vi "2023_day08_Task2.vi"() -> ()   [LabVIEW 2021]
panel:
  out "Task 2":u64
  in  "Switch":bool caption="Ex. Data  vs.  User Data"
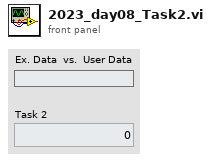
[diagram p1: front panel]
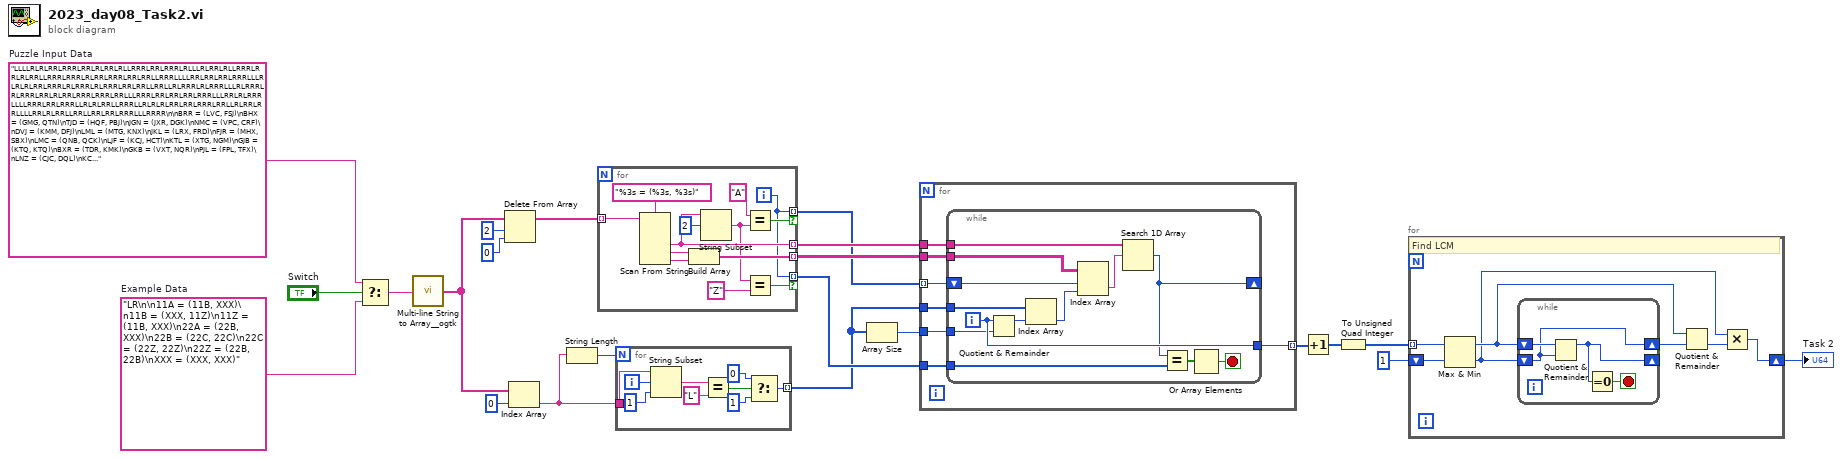
[diagram p0: block diagram]
diagram:
  w21 = "LLLLRLRLRRLRRRLRRLRLRRLRLLRRRLRRLRRRLRLLLRLRRLRLLRRRLRRLRLRRLLRRRLRRRLRLRRLRRRLRRLRRLLRRRLLLLRRLRRLRRLRRRLLLRLRLRLRRLRRRLRLRRRLRLRRRLRRLRRLLRRLLRLRRRLRLRRRLLLRLRRRLRLRRRLRRLRLRRLRRRLRRRLRRLLLRRRLRRLRRLRRLRRRLLLRRLRLRRRLLLLRRRLRRLRRRLLRLRLRRLLRRRLLRLRLRLRRLRRLRRRLRRLLRLRRLRRLLLLRRLRLRRLLRRLLRRLRRLRRRLLLRRRR\n\nBRR = (LVC, FSJ)\nBHX = (GMG, QTN)\nTJD = (HQF, PBJ)\nJGN = (JXR, DGK)\nNMC = (VPC, CRF)\nDVJ = (KMM, DFJ)\nLML = (MTG, KNX)\nJKL = (LRX, FRD)\nFJR = (MHX, SBX)\nLMC = (QNB, QCK)\nLJF = (KCJ, HCT)\nKTL = (XTG, NGM)\nGJB = (KTQ, KTQ)\nBXR = (TDR, KMK)\nGKB = (VXT, NQR)\nPJL = (FPL, TFX)\nLNZ = (CJC, DQL)\nKCG = (KDL, LMF)\nPGG = (NDL, XXC)\nPMS = (XQM, DFG)\nCJF = (MCG, RTJ)\nJTH = (PGS, SGZ)\nQBS = (JSC, KMT)\nDQL = (KRR, PBL)\nHSF = (SNP, KJR)\nXVQ = (VQR, HSX)\nQKF = (PBT, XLC)\nDNA = (DQL, CJC)\nLNF = (RVC, TJD)\nMKT = (LDX, CGC)\nBXP = (RGX, TTR)\nSBX = (PGT, JGN)\nJQK = (HDQ, BHQ)\nMHL = (TLX, JDN)\nBBD = (QNJ, BRM)\nMTT = (BVK, DXB)\nFVR = (VLN, PRV)\nRVC = (HQF, PBJ)\nLDX = (LRS, KBV)\nBKF = (PXH, TNB)\nBRM = (XTV, NGH)\nDDL = (JNG, SFF)\nBBT = (BQJ, BCN)\nGPK = (CVK, DDL)\nTLX = (BDN, XNT)\nJHL = (BRX, QBT)\nNTL = (HSR, DJD)\nXBH = (PJX, JQK)\nPPF = (LCT, BJL)\nSFF = (FVR, NFG)\nHNA = (CTC, BSG)\nCNG = (DXM, QFN)\nGML = (NRD, TVN)\nRHH = (NBT, LJH)\nLDM = (DDN, TRN)\nXSK = (PLB, NVJ)\nNCQ = (MDN, XGT)\nFCQ = (HCT, KCJ)\nDRC = (JKL, JNM)\nSHR = (KLX, VLH)\nFTP = (DRN, DKV)\nQBF = (GVS, NXK)\nGXK = (XDK, LVF)\nKMK = (VXV, XCS)\nPKK = (QNJ, BRM)\nNJH = (TKL, PQK)\nBRX = (MNM, HVC)\nVTD = (BJK, LML)\nQVX = (DVJ, DSF)\nGRM = (JCV, SQB)\nRDQ = (HCG, XMB)\nRGX = (FCN, TPD)\nHBH = (FPR, DHX)\nPHM = (JSP, RCR)\nNBT = (FRG, CMJ)\nXRH = (HCB, FBM)\nGMR = (FDJ, NJD)\nMVG = (RDJ, QSD)\nBDL = (JSB, TFN)\nVXT = (MBM, JND)\nTXC = (QDG, LTV)\nSRL = (RRX, NDS)\nSGN = (MPL, CBB)\nHVH = (SLJ, CBC)\nVPC = (CCG, QSJ)\nKCJ = (CKC, TTD)\nRLT = (LLT, VVL)\nRXV = (KXQ, VBR)\nFQS = (STP, BHX)\nSGC = (RLJ, QGB)\nXLX = (HRG, DGV)\nXKV = (QQB, TNQ)\nSLJ = (GTB, MPF)\nPKV = (CQN, THS)\nRPP = (QFT, TNK)\nDKL = (MFC, MFC)\nBCG = (FXM, GPR)\nRFV = (DRC, MPD)\nVVC = (FGN, CVL)\nHQB = (QNT, VVC)\nRRP = (VVC, QNT)\nTRS = (RCM, GHN)\nQBT = (HVC, MNM)\nXKS = (SCC, VXX)\nTPS = (FMH, KFN)\nMTS = (VXT, NQR)\nFXM = (LDM, FQT)\nLNB = (XJV, SJN)\nHVF = (QXC, RBH)\nLSG = (QHM, TSM)\nJMP = (HBH, NQK)\nNGM = (KDP, HHP)\nHCG = (SLR, TSC)\nHGX = (DFG, XQM)\nDLG = (BVN, GMM)\nDJD = (VGP, VML)\nHBT = (XKL, JBQ)\nNVJ = (GKX, PKS)\nCPS = (PKJ, RSV)\nSKN = (NBT, LJH)\nCCK = (TTJ, SLV)\nDXM = (CBN, BXR)\nRJD = (XJH, SKH)\nRDJ = (CNF, TTG)\nPKJ = (BCM, XKC)\nFQL = (SRV, DFC)\nKDS = (MFB, CLQ)\nQKR = (VGD, CXK)\nXXC = (NFD, SPS)\nPSQ = (NJH, BLR)\nBLR = (PQK, TKL)\nLMX = (DGV, HRG)\nGCK = (CSR, CSR)\nGKJ = (JHL, PNN)\nGVS = (TLN, LJX)\nFPR = (JCH, GKD)\nVQV = (DGB, GGN)\nCPF = (VMH, JQQ)\nGKD = (SGF, PHM)\nJNM = (LRX, FRD)\nCXV = (LNF, HGF)\nTNK = (RRD, HKC)\nDXX = (LMC, ZZZ)\nDGG = (PPF, TRR)\nMLH = (TVL, PBR)\nLBC = (LJL, FTR)\nFVQ = (TBC, LKB)\nLTF = (CBC, SLJ)\nTVH = (XMS, GJS)\nSFB = (TTJ, SLV)\nLVF = (MBT, SJB)\nXPP = (QDM, PJL)\nBVK = (RPV, JMP)\nVGD = (MRX, FJR)\nFRD = (XBH, CDN)\nLKM = (CMF, XNS)\nTCJ = (MMS, PGG)\nDHQ = (MTT, BKS)\nHDQ = (GPH, XKH)\nKTJ = (QQT, MKR)\nNMQ = (VFK, VSD)\nRSK = (QDM, PJL)\nXQC = (KFP, HVB)\nLQN = (NGM, XTG)\nTKG = (XDQ, XDQ)\nKBB = (VQR, HSX)\nTQQ = (QDG, LTV)\nSQN = (TDQ, XKV)\nTSM = (TSH, MRP)\nKPH = (THS, CQN)\nHCB = (DVL, RTV)\nMLR = (GHT, NSN)\nBFM = (GCK, SLX)\nGXQ = (QKM, JJL)\nGNF = (HRQ, XTK)\nTRR = (BJL, LCT)\nAAA = (QNB, QCK)\nSDL = (KJX, LSN)\nDKV = (KBB, XVQ)\nRMR = (MQR, CPR)\nMQC = (CBV, SRP)\nPRV = (KDS, FBX)\nGTB = (CCK, SFB)\nSNP = (PXX, SHR)\nNTR = (VHT, KXK)\nMKJ = (DDL, CVK)\nLSQ = (HSF, RMN)\nTTJ = (CBH, QKF)\nDNH = (MVG, JCJ)\nKMM = (KPH, PKV)\nNTT = (RQK, PFK)\nQMF = (BFM, PJB)\nRJB = (RBH, QXC)\nLRS = (MJT, BVM)\nCJG = (RMR, BMN)\nDVQ = (GXM, DDH)\nMFC = (LMC, LMC)\nXTG = (HHP, KDP)\nHKB = (RDQ, TVT)\nPKS = (JQM, DGG)\nBJK = (KNX, MTG)\nTVT = (XMB, HCG)\nJNR = (JHG, JLN)\nVFK = (XKS, QBH)\nNPC = (PKK, BBD)\nPXX = (KLX, VLH)\nXLC = (NST, BXP)\nCBB = (LMX, XLX)\nKLX = (MSH, LCF)\nCLQ = (JNF, JNC)\nTSS = (MKR, QQT)\nSSS = (RMQ, RCS)\nQSD = (TTG, CNF)\nNHG = (DVQ, VNB)\nCTC = (VCN, RJD)\nTHS = (QRH, GPT)\nKDR = (RTK, GKJ)\nNTD = (CGG, SPN)\nGHP = (NCQ, FCD)\nKXQ = (RLS, VRM)\nGNV = (BQJ, BCN)\nDXQ = (QHC, FXN)\nRQB = (FVQ, TNF)\nCNF = (TXC, TQQ)\nBGB = (QQS, LRV)\nZZZ = (QCK, QNB)\nNFM = (MGV, VTD)\nMFD = (DBF, KSN)\nNST = (RGX, TTR)\nXJV = (LGL, LGL)\nTRQ = (TVH, KJL)\nPPV = (CJP, VHH)\nDNV = (DBM, VGJ)\nJBQ = (MHL, RFN)\nHRG = (JFD, VQP)\nRMB = (JKJ, JGJ)\nRGQ = (RSK, XPP)\nKHF = (TJG, KPX)\nHPZ = (BSG, CTC)\nLFJ = (TSN, NMB)\nMBT = (XRC, PJR)\nQFN = (CBN, BXR)\nQSJ = (BRS, BKF)\nXJH = (RSF, VNP)\nGST = (LVF, XDK)\nDDN = (NMS, RLT)\nCXK = (FJR, MRX)\nPHH = (FPB, TCJ)\nXHV = (KTJ, TSS)\nVHT = (NPC, DMG)\nRNL = (NHG, DVN)\nTKL = (KPN, FKX)\nDGB = (GPJ, QMF)\nPNN = (QBT, BRX)\nTBC = (NTR, FKG)\nPGS = (QDT, JQL)\nSLX = (CSR, LNB)\nBVV = (LVC, FSJ)\nJQL = (MLH, GSC)\nPXH = (CJF, CKM)\nLHM = (DSF, DVJ)\nNND = (NTD, DTB)\nMFB = (JNF, JNC)\nTTR = (FCN, TPD)\nHRQ = (JTD, JTD)\nSLR = (TXT, JSN)\nVQP = (XPK, XGB)\nQHM = (MRP, TSH)\nRTJ = (PXB, TLP)\nQQT = (RRL, QHQ)\nCSR = (XJV, XJV)\nCJP = (CJG, HQQ)\nRMC = (MPD, DRC)\nXMS = (LXX, GPN)\nHSR = (VGP, VML)\nMNM = (VSS, QXR)\nSJN = (LGL, LNZ)\nKBV = (MJT, BVM)\nKFN = (NRC, VSG)\nJNC = (RHR, LFJ)\nMPF = (SFB, CCK)\nQVK = (GNK, BCG)\nNJD = (KCG, LDB)\nDBM = (MJG, MFD)\nNKF = (GGN, DGB)\nBCN = (JNR, MHK)\nGNK = (FXM, GPR)\nKMT = (HFC, CPS)\nFDJ = (KCG, LDB)\nLVD = (PHH, QDR)\nFCN = (VDP, MQC)\nQQB = (GJB, GJB)\nPLF = (JNL, HBT)\nQDM = (FPL, TFX)\nGXM = (CLD, NNL)\nMRV = (BCG, GNK)\nLKB = (NTR, FKG)\nTTG = (TQQ, TXC)\nGFD = (VSD, VFK)\nRCS = (KQQ, DNH)\nQXR = (FCQ, LJF)\nHMQ = (RJQ, FQL)\nVCN = (SKH, XJH)\nQQG = (HSR, DJD)\nHGF = (RVC, TJD)\nXMB = (TSC, SLR)\nPJB = (GCK, SLX)\nHFC = (RSV, PKJ)\nJJL = (GXK, GST)\nQTN = (JLV, SGX)\nKDP = (GNV, BBT)\nVRF = (TFN, JSB)\nGPN = (CPF, SRQ)\nTSC = (TXT, JSN)\nCRF = (QSJ, CCG)\nTNF = (TBC, LKB)\nVLH = (LCF, MSH)\nBCV = (JSC, KMT)\nNNL = (KVX, FQS)\nRVT = (HCB, FBM)\nQHC = (QKV, NCJ)\nVDP = (CBV, SRP)\nCBV = (VQV, NKF)\nCMF = (XHV, TPR)\nTRN = (RLT, NMS)\nJSB = (XTH, TRS)\nCFC = (TVT, RDQ)\nKDL = (TKG, TKG)\nTTD = (BBC, GHP)\nKJR = (PXX, SHR)\nMTV = (GVS, NXK)\nBVN = (KDR, PVP)\nDXB = (RPV, JMP)\nFSJ = (QPQ, GML)\nPBJ = (LQN, KTL)\nPXB = (BDL, VRF)\nNDS = (BGB, NGX)\nCBN = (KMK, TDR)\nNFG = (VLN, PRV)\nJTD = (PGS, PGS)\nMKR = (QHQ, RRL)\nJSN = (RFV, RMC)\nCVK = (SFF, JNG)\nFGN = (BVQ, XQC)\nHHF = (RPS, QQF)\nPLB = (PKS, GKX)\nBJB = (QMC, GPG)\nSTP = (QTN, GMG)\nDGK = (RKK, BVT)\nJJM = (VGD, CXK)\nLTS = (QPN, BCL)\nLVC = (QPQ, GML)\nQNB = (GJN, RVB)\nRBH = (HMQ, HPS)\nNQK = (DHX, FPR)\nMRP = (BDT, SGN)\nJQM = (TRR, PPF)\nTSH = (BDT, SGN)\nJLN = (JCC, FCB)\nBRP = (LDX, CGC)\nSJC = (HRQ, HRQ)\nLJL = (BVB, PPV)\nSPN = (SDL, VHM)\nSDM = (DDF, LTS)\nLJH = (FRG, CMJ)\nCMG = (MKD, JGT)\nGPR = (LDM, FQT)\nQPQ = (NRD, TVN)\nJCJ = (RDJ, QSD)\nHSX = (CMG, SHF)\nVML = (RMB, MHC)\nDHX = (JCH, GKD)\nMTG = (FPX, SPD)\nBDT = (MPL, CBB)\nCJC = (PBL, KRR)\nJLS = (LJL, FTR)\nHQF = (LQN, KTL)\nHQQ = (RMR, BMN)\nQMC = (RBP, PXD)\nRPV = (HBH, NQK)\nJHG = (JCC, FCB)\nTPD = (VDP, MQC)\nBHQ = (XKH, GPH)\nXKC = (HDD, GXR)\nRPS = (KJP, KJP)\nQNT = (CVL, FGN)\nJSC = (HFC, CPS)\nKXG = (DTB, NTD)\nCKM = (RTJ, MCG)\nFTD = (KPX, TJG)\nVSD = (XKS, QBH)\nMCG = (TLP, PXB)\nXKH = (HLP, CXV)\nTNB = (CJF, CKM)\nXTH = (RCM, GHN)\nDFN = (GMR, DSS)\nLMF = (TKG, XST)\nFMH = (NRC, VSG)\nXCS = (JTS, GRM)\nGVF = (NDS, RRX)\nCXM = (HGX, PMS)\nVRM = (XJT, DXQ)\nJLV = (QVX, LHM)\nJCH = (PHM, SGF)\nNMS = (VVL, LLT)\nBHS = (XJR, LKM)\nCKC = (BBC, GHP)\nCBH = (XLC, PBT)\nPRL = (QFT, TNK)\nSDF = (VTD, MGV)\nRVB = (MLR, XHT)\nGPT = (PLF, MJX)\nKRR = (RVT, XRH)\nGXR = (BVV, BRR)\nNSN = (RGQ, JMQ)\nKJX = (TCR, MSL)\nPHL = (TSM, QHM)\nMQR = (MTS, GKB)\nXDK = (SJB, MBT)\nNRC = (DGN, BJB)\nJQQ = (LBC, JLS)\nJTS = (JCV, SQB)\nRLJ = (JJM, QKR)\nDTB = (CGG, SPN)\nBRS = (PXH, TNB)\nSRV = (SPC, DNV)\nMNP = (JJL, QKM)\nKTQ = (XSK, XSK)\nFPX = (SJC, GNF)\nVBR = (VRM, RLS)\nKSN = (HQB, RRP)\nRJQ = (SRV, DFC)\nBKS = (BVK, DXB)\nBVB = (VHH, CJP)\nXTK = (JTD, JTH)\nPBT = (BXP, NST)\nPVP = (RTK, GKJ)\nQPN = (BCV, QBS)\nQQF = (KJP, HPZ)\nQRH = (PLF, MJX)\nGHS = (BKN, TPS)\nRCM = (MNP, GXQ)\nDCT = (DDF, LTS)\nJLC = (HGX, PMS)\nVNC = (XSK, CXZ)\nBQJ = (MHK, JNR)\nSHF = (JGT, MKD)\nFXN = (QKV, NCJ)\nFPB = (PGG, MMS)\nJGJ = (KXG, NND)\nVBM = (PSQ, QKN)\nGKX = (DGG, JQM)\nDSF = (KMM, DFJ)\nCMJ = (GPK, MKJ)\nNCJ = (SDM, DCT)\nMKD = (GQG, DHQ)\nCFZ = (RQB, SHH)\nRQK = (DKL, DKL)\nXGT = (HPQ, VRQ)\nSRP = (NKF, VQV)\nBSG = (VCN, RJD)\nXRC = (NFM, SDF)\nDVL = (SRL, GVF)\nHVB = (HXS, MLD)\nMPD = (JNM, JKL)\nJSP = (PHL, LSG)\nBCR = (XJR, LKM)\nPQK = (KPN, FKX)\nFCD = (XGT, MDN)\nMDL = (JLC, CXM)\nFBX = (CLQ, MFB)\nVNP = (RGM, GHS)\nHMK = (RMN, HSF)\nSJB = (PJR, XRC)\nJFD = (XPK, XGB)\nHHP = (GNV, BBT)\nTVN = (VBM, KJN)\nDMG = (PKK, BBD)\nRGM = (BKN, TPS)\nTRF = (KXQ, VBR)\nXHT = (NSN, GHT)\nDFJ = (KPH, PKV)\nKJP = (CTC, BSG)\nLLT = (NTS, LVD)\nRMN = (SNP, KJR)\nGSC = (TVL, PBR)\nRSV = (XKC, BCM)\nTLP = (VRF, BDL)\nGGN = (GPJ, QMF)\nXJR = (CMF, XNS)\nGQG = (BKS, MTT)\nJPN = (MRV, QVK)\nRSF = (RGM, GHS)\nQQS = (DLG, JPV)\nDGV = (VQP, JFD)\nJDN = (XNT, BDN)\nLMA = (QDT, JQL)\nQDG = (QGC, DTX)\nHDD = (BVV, BRR)\nRRD = (CNG, XLJ)\nQBH = (VXX, SCC)\nGPH = (HLP, CXV)\nCVN = (MRV, QVK)\nRLS = (XJT, DXQ)\nQKN = (NJH, BLR)\nNRD = (VBM, KJN)\nNMB = (HVF, RJB)\nXNT = (RXV, TRF)\nXNS = (XHV, TPR)\nSGX = (LHM, QVX)\nNTS = (PHH, QDR)\nSPS = (LTF, HVH)\nKPX = (BCR, BHS)\nGNM = (RPS, RPS)\nCXZ = (NVJ, PLB)\nVVL = (LVD, NTS)\nVTC = (NHG, DVN)\nPXD = (BHH, SSS)\nTVL = (MKT, BRP)\nTPR = (KTJ, TSS)\nMJX = (JNL, HBT)\nBKN = (FMH, KFN)\nMBM = (BVC, FTP)\nRTV = (GVF, SRL)\nGPG = (PXD, RBP)\nKXK = (DMG, NPC)\nJPV = (GMM, BVN)\nLXP = (VPC, CRF)\nRMQ = (DNH, KQQ)\nDRN = (KBB, XVQ)\nMMS = (XXC, NDL)\nGMG = (SGX, JLV)\nMJT = (KHF, FTD)\nXJT = (QHC, FXN)\nJMQ = (XPP, RSK)\nQCS = (TVH, KJL)\nBVC = (DRN, DKV)\nSPC = (DBM, VGJ)\nSHH = (TNF, FVQ)\nVGA = (PLB, NVJ)\nRKK = (JPN, CVN)\nSCC = (TRQ, QCS)\nCDN = (JQK, PJX)\nVSS = (LJF, FCQ)\nJNF = (LFJ, RHR)\nVGP = (MHC, RMB)\nVGJ = (MJG, MFD)\nQGC = (RHH, SKN)\nRKJ = (KTQ, VNC)\nDTX = (SKN, RHH)\nHPQ = (VDR, SGC)\nCCG = (BRS, BKF)\nVLN = (FBX, KDS)\nBHH = (RMQ, RCS)\nBBC = (FCD, NCQ)\nJCV = (GNM, GNM)\nTNQ = (GJB, RKJ)\nQNJ = (NGH, XTV)\nGHT = (RGQ, JMQ)\nLJX = (CFC, HKB)\nTLN = (HKB, CFC)\nPFK = (DKL, LFL)\nPJR = (SDF, NFM)\nJNG = (NFG, FVR)\nPJX = (BHQ, HDQ)\nVHH = (CJG, HQQ)\nRTK = (PNN, JHL)\nXGB = (MLN, SQN)\nJCC = (NQX, NTT)\nBVT = (CVN, JPN)\nHPS = (RJQ, FQL)\nTCR = (DFN, RHS)\nLLA = (SHH, RQB)\nNGX = (QQS, LRV)\nSLV = (CBH, QKF)\nBMN = (CPR, MQR)\nXKL = (RFN, MHL)\nCGG = (VHM, SDL)\nKJN = (PSQ, QKN)\nLDB = (KDL, LMF)\nSPD = (SJC, GNF)\nVDR = (RLJ, QGB)\nDDF = (QPN, BCL)\nKQQ = (MVG, JCJ)\nDSS = (FDJ, NJD)\nNFD = (HVH, LTF)\nGPJ = (BFM, PJB)\nLGL = (DQL, CJC)\nTDQ = (QQB, TNQ)\nRCR = (PHL, LSG)\nSKH = (VNP, RSF)\nDGN = (QMC, GPG)\nNGH = (RNL, VTC)\nTSN = (HVF, RJB)\nMGV = (LML, BJK)\nQHQ = (LXP, NMC)\nKJL = (GJS, XMS)\nRBP = (BHH, SSS)\nQDR = (FPB, TCJ)\nRHR = (NMB, TSN)\nNXK = (LJX, TLN)\nFCB = (NQX, NTT)\nTFN = (TRS, XTH)\nMJG = (KSN, DBF)\nBVQ = (KFP, HVB)\nGMM = (PVP, KDR)\nMDN = (VRQ, HPQ)\nLTV = (DTX, QGC)\nLRV = (DLG, JPV)\nMHC = (JKJ, JGJ)\nDFC = (DNV, SPC)\nLXV = (SHH, RQB)\nPBL = (RVT, XRH)\nBDN = (RXV, TRF)\nJKJ = (KXG, NND)\nMSH = (MTV, QBF)\nNDL = (SPS, NFD)\nFKG = (VHT, KXK)\nPBR = (MKT, BRP)\nVSG = (BJB, DGN)\nRRX = (BGB, NGX)\nNQR = (JND, MBM)\nMRX = (MHX, SBX)\nDVN = (DVQ, VNB)\nHKC = (CNG, XLJ)\nPGT = (JXR, DGK)\nDBF = (HQB, RRP)\nFRG = (GPK, MKJ)\nDFG = (NMQ, GFD)\nQDT = (MLH, GSC)\nKVX = (STP, BHX)\nLCT = (MDL, KCL)\nLSN = (TCR, MSL)\nTXT = (RMC, RFV)\nMXM = (LXV, CFZ)\nTJG = (BHS, BCR)\nBCM = (GXR, HDD)\nFKX = (NTL, QQG)\nSRQ = (JQQ, VMH)\nBCL = (BCV, QBS)\nLRX = (CDN, XBH)\nRHS = (DSS, GMR)\nCLD = (FQS, KVX)\nXLJ = (DXM, QFN)\nKCL = (CXM, JLC)\nHXS = (PRL, RPP)\nJND = (BVC, FTP)\nVQR = (SHF, CMG)\nVNB = (DDH, GXM)\nQGB = (JJM, QKR)\nCVL = (BVQ, XQC)\nRFN = (JDN, TLX)\nFBM = (DVL, RTV)\nTFX = (LSQ, HMK)\nXQM = (NMQ, GFD)\nBJL = (KCL, MDL)\nFTR = (PPV, BVB)\nKNX = (FPX, SPD)\nMHK = (JHG, JLN)\nTDR = (XCS, VXV)\nHVC = (VSS, QXR)\nQXC = (HPS, HMQ)\nRRL = (NMC, LXP)\nMLD = (PRL, RPP)\nLCF = (MTV, QBF)\nVXV = (JTS, GRM)\nXTV = (RNL, VTC)\nLFL = (MFC, DXX)\nCBC = (GTB, MPF)\nCQN = (GPT, QRH)\nDDH = (NNL, CLD)\nGHN = (GXQ, MNP)\nJGT = (DHQ, GQG)\nHCT = (CKC, TTD)\nQCK = (GJN, RVB)\nSGF = (JSP, RCR)\nMPL = (XLX, LMX)\nXDQ = (LXV, LXV)\nMLN = (TDQ, XKV)\nSGZ = (JQL, QDT)\nVRQ = (SGC, VDR)\nFPL = (LSQ, HMK)\nSQB = (GNM, HHF)\nMHX = (PGT, JGN)\nQFT = (HKC, RRD)\nLXX = (CPF, SRQ)\nCPR = (GKB, MTS)\nHLP = (LNF, HGF)\nGJS = (GPN, LXX)\nQKV = (DCT, SDM)\nXST = (XDQ, MXM)\nVXX = (QCS, TRQ)\nKFP = (HXS, MLD)\nMSL = (RHS, DFN)\nNQX = (RQK, PFK)\nCGC = (LRS, KBV)\nFQT = (TRN, DDN)\nVMH = (LBC, JLS)\nVHM = (LSN, KJX)\nJXR = (BVT, RKK)\nKPN = (QQG, NTL)\nQKM = (GST, GXK)\nJNL = (XKL, JBQ)\nBVM = (KHF, FTD)\nXPK = (SQN, MLN)\nGJN = (MLR, XHT)"  # Puzzle Input Data
  w7 = "LR\n\n11A = (11B, XXX)\n11B = (XXX, 11Z)\n11Z = (11B, XXX)\n22A = (22B, XXX)\n22B = (22C, 22C)\n22C = (22Z, 22Z)\n22Z = (22B, 22B)\nXXX = (XXX, XXX)"  # Example Data
  n1 = Select(t=w21, s="Switch", f=w7) -> (s? t:f=w20:string)
  n2 = call <userlib>:"Multi-line String to Array__ogtk.vi"("string"=w20) -> ("lines"=w17:string[])
  n3 = Delete From Array(array=w17, length=2, index=0) -> (array with subset deleted=w13:string[])  [unwired: 1 out]
  n4 = Index Array(array=w17, index=0) -> (element=w15:string)
  n5 = String Length(string=w15) -> (length=w14:i32)
  n6 = for {
    tunnel: w13 -> [w35] mode=indexing
    tunnel: [w34] -> w11 mode=indexing
    tunnel: [w28] -> w12 mode=indexing
    tunnel: [w24] -> w10 mode=indexing if=w27
    tunnel: [w24] -> w6 mode=indexing if=w23
    i -> [w24]
    n7 = Scan From String(format string="%3s = (%3s, %3s)", input string=w35) -> (output 1=w28:string, output 2=w31:string, output 3=w32:string)  [unwired: 5 in, 3 out]
    n8 = Build Array(w31, w32) -> (w34:string[])
    n9 = String Subset(string=w28, offset (0)=2) -> (substring=w25:string)  [unwired: 1 in]
    n10 = Equal?(x="A", y=w25) -> (x = y?=w27:bool)
    n11 = Equal?(x=w25, y="Z" ("x")) -> (x = y?=w23:bool)
  }
  n12 = for {
    N: w14 -> [_]
    tunnel: w15 -> [w44]
    tunnel: [w37] -> w5 mode=indexing
    i -> [w43]
    n13 = String Subset(string=w44, offset (0)=w43, length (rest)=1 ("length (rest)")) -> (substring=w38:string)
    n14 = Equal?(x=w38, y="L") -> (x = y?=w36:bool)
    n15 = Select(t=0, s=w36, f=1) -> (s? t:f=w37:i32)
  }
  n16 = Array Size(array=w5) -> (size(s)=w9:i32)
  n17 = for {
    tunnel: w12 -> [w51]
    tunnel: w11 -> [w50]
    tunnel: w10 -> [w49] mode=indexing
    tunnel: w5 -> [w48]
    tunnel: w9 -> [w47]
    tunnel: [w45] -> w8 mode=indexing
    tunnel: w6 -> [w46]
    n18 = while {
      tunnel: w48 -> [w64]
      tunnel: w51 -> [w62]
      tunnel: w50 -> [w60]
      shift-right: [w55] -> _
      shift-left: w49 -> [w59]
      tunnel: [w58] -> w45
      tunnel: w47 -> [w57]
      tunnel: w46 -> [w52]
      i -> [w58]
      stop <- w53 stop-if-true
      n19 = Quotient & Remainder(x=w58, y=w57) -> (x-y*floor(x/y)=w63:i32)  [unwired: 1 out]
      n20 = Index Array(array=w64, index=w63) -> (element=w61:i32)
      n21 = Index Array(array=w60, index (row)=w59, index (col)=w61) -> (element=w56:string)
      n22 = Search 1D Array(1D array=w62, element=w56) -> (index of element=w55:i32)  [unwired: 1 in]
      n23 = Equal?(x=w55, y=w52) -> (x = y?=w54:bool[])
      n24 = Or Array Elements(Boolean array=w54) -> (logical OR=w53:bool)
    }
  }
  n25 = Increment(x=w8) -> (x+1=w4:i32[])
  n26 = To Unsigned Quad Integer(1:w4) -> (0:w3:u64[])
  n27 = for {
    tunnel: w3 -> [w70] mode=indexing
    shift-right: [w65] -> w1
    shift-left: u64 1 -> [w71]
    # "Find LCM"
    n28 = Max & Min(x=w70, y=w71) -> (max(x,y)=w68:u64, min(x,y)=w67:u64)
    n29 = while {
      shift-right: [w73] -> w69
      shift-left: w68 -> [w75]
      shift-right: [w72] -> _
      shift-left: w67 -> [w73]
      stop <- w74 stop-if-true
      n30 = Quotient & Remainder(x=w75, y=w73) -> (x-y*floor(x/y)=w72:u64)  [unwired: 1 out]
      n31 = Equal To 0?(x=w72) -> (x = 0?=w74:bool)
    }
    n32 = Quotient & Remainder(x=w68, y=w69) -> (floor(x/y)=w66:u64)  [unwired: 1 out]
    n33 = Multiply(x=w67, y=w66) -> (x*y=w65:u64)
  }
  "Task 2" <- w1
